vi "Register Reflection Descriptors.vi"(8 "error in":errorcluster, 10 "reflector description strings":string[](array[string]), 11 "gRPCid in":T1) -> (0 "error out":errorcluster, 3 "gRPCid out":T1)   [LabVIEW 2019, in "grpc-lvsupport.lvlib"]
uses:
  grpc-lvsupport.lvlib
  Shared/grpcId.ctl
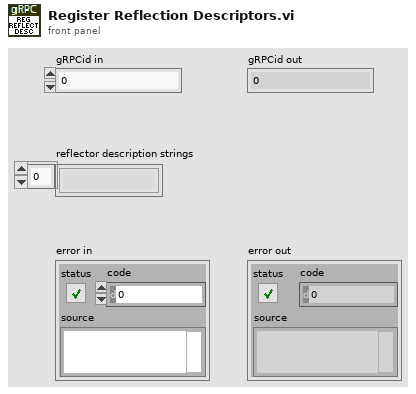
[diagram p1: front panel]
types:
  T1 = typedef "grpc-lvsupport.lvlib/grpcId.ctl" = u64
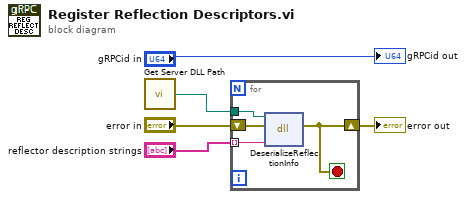
[diagram p0: block diagram]
diagram:
  n1 = call "Get Server DLL Path.vi"() -> ("server dll path"=w4:path)
  n2 = for {
    tunnel: w4 -> [w9]
    tunnel: "reflector description strings" -> [w8] mode=indexing
    shift-right: [w6] -> w5
    shift-left: "error in" -> [w7]
    stop <- w6 stop-if-true
    n3 = dll-call lib="?" fn="DeserializeReflectionInfo"(path in=w9, error in=w7, "serializedDescriptor"=w8) -> (error out=w6:errorcluster)  [unwired: 3 in, 1 out]
  }
  "error out" <- w5
  "gRPCid out" <- "gRPCid in"
